vi "Erase (single).vi"(8 "error in (no error)":errorcluster, 10 "Key":string, 11 "Parameter to Hardware Map in":refnum<class "Parameter to Hardware Map.lvclass">) -> (0 "error out":errorcluster, 2 "Deleted Pair":T1, 3 "Parameter to Hardware Map out":refnum<class "Parameter to Hardware Map.lvclass">)   [LabVIEW 2020, in "RxnRover.lvlib" / "Parameter to Hardware Map.lvclass"]
doc: "Removes the element from the map specified by the given key."
uses:
  Parameter to Hardware Map.lvclass
  Pair.ctl
  Controller/Generic Plugin.lvclass
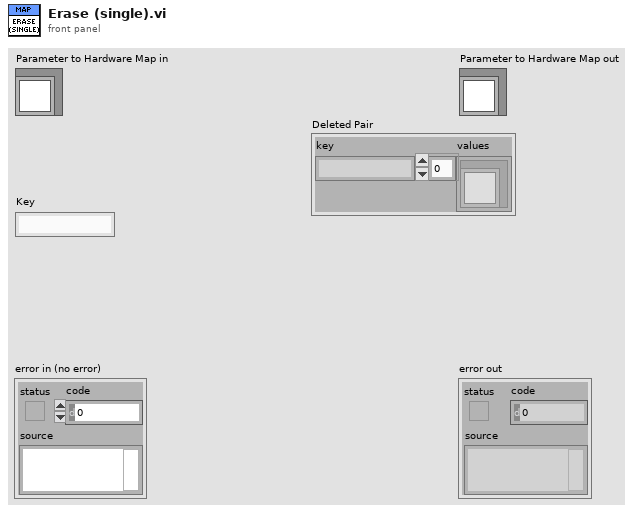
[diagram p1: front panel]
types:
  T1 = typedef "RxnRover.lvlib/Parameter to Hardware Map.lvclass/Pair.ctl" = cluster{"key":string, "values":refnum<class "Generic Plugin.lvclass">[]}
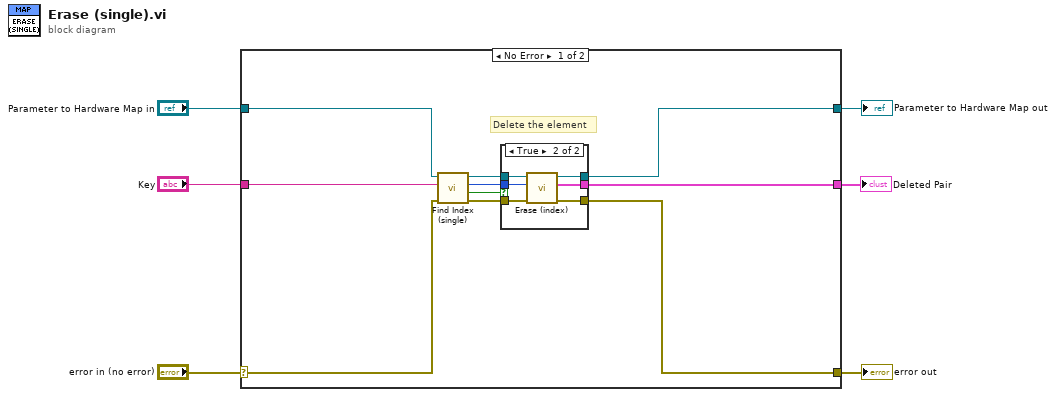
[diagram p0: block diagram]
diagram:
  n1 = case shown="No Error" "error in (no error)" {
    selector: "error in (no error)" -> [w14 w26]
    tunnel: [w8 w26] -> w5
    tunnel: [w9 w25] -> w3
    tunnel: "Parameter to Hardware Map in" -> [w16 w25]
    tunnel: "Key" -> [w15 _]
    tunnel: [w7 _] -> w1
    frame No Error {
      # "Delete the element"
      n2 = call "Find Index (single).vi"("error in (no error)"=w14, "Key"=w15, "Parameter to Hardware Map in"=w16) -> ("error out"=w13:errorcluster, "Found?"=w10:bool, "Index"=w11:i32, "Parameter to Hardware Map out"=w12:refnum<class "Parameter to Hardware Map.lvclass">)  [unwired: 5 in]
      n3 = case shown="True" w10 {
        tunnel: w13 -> [w17 w24]
        tunnel: w12 -> [w18 w23]
        tunnel: w11 -> [_ w22]
        tunnel: [w18 w21] -> w9
        tunnel: [w17 w20] -> w8
        tunnel: [_ w19] -> w7
        frame False {
        }
        frame True {
          n4 = call "Erase (index).vi"("error in (no error)"=w24, "Index"=w22, "Parameter to Hardware Map in"=w23) -> ("error out"=w20:errorcluster, "Deleted Pair"=w19:T1, "Parameter to Hardware Map out"=w21:refnum<class "Parameter to Hardware Map.lvclass">)  [unwired: 6 in]
        }
      }
    }
    frame Error {
    }
  }
  "error out" <- w5
  "Parameter to Hardware Map out" <- w3
  "Deleted Pair" <- w1
